vi "dfd_C Build Output File Paths.vi"(10 "destination folder":path, 11 "filter name":string) -> (1 "typedef path":path, 2 "H path":path, 3 "C path":path)   [LabVIEW 2017, in "NI_DigFilterLicensed.lvlib"]
uses:
  <vilib>/addons/Digital Filter Design/NI_DigFilterLicensed.lvlib
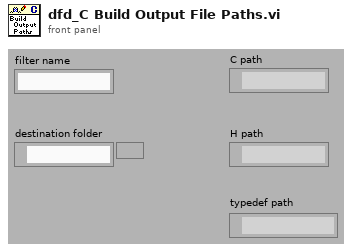
[diagram p1: front panel]
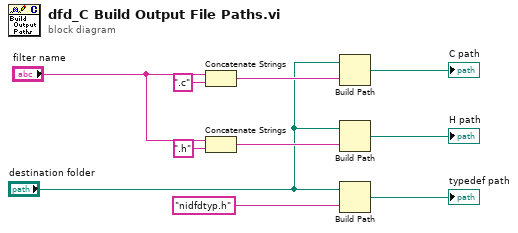
[diagram p0: block diagram]
diagram:
  n1 = Concatenate Strings("filter name", ".c" ("string")) -> (w4:string)
  n2 = Concatenate Strings("filter name", ".h" ("string")) -> (w10:string)
  n3 = Build Path(base path="destination folder", name or relative path=w4) -> (appended path=→"C path":path)
  n4 = Build Path(base path="destination folder", name or relative path=w10) -> (appended path=→"H path":path)
  n5 = Build Path(base path="destination folder", name or relative path="nidfdtyp.h") -> (appended path=→"typedef path":path)
